vi "Read Digital channels.vi"   [LabVIEW 2020, in "BDAQ-6104.lvlib"]
uses:
  <instrlib>/BDAQ-6104/BDAQ-6104.lvlib
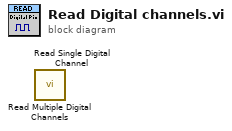
[diagram p0: block diagram]
diagram:
  n1 = call <instrlib>:"Read Multiple Digital Channels.vi"() -> ()  [unwired: 9 in, 3 out]
  n2 = call <instrlib>:"Read Single Digital Channel.vi"() -> ()  [unwired: 9 in, 3 out]
